vi "read can fd.vi"(8 "error in (no error)":errorcluster, 11 "channel":u16 format="%x") -> (0 "error out":errorcluster, 2 "queue empty?":bool, 3 "message":T5 {"id" format="%x"; "data" format="%x"}, 5 "ecc register":T1)   [LabVIEW 2024, in "atsj peakcan basic.lvlib"]
doc: "Reads a CAN FD message from the receive queue of an FD-capable PeakCAN <b>channel</b>."
uses:
  atsj peakcan basic.lvlib
  message type.ctl
  message.ctl
  support/x64/PCANBasic.dll
  ecc register error code.ctl
  ecc register direction.ctl
  ecc register segment.ctl
  ecc register.ctl
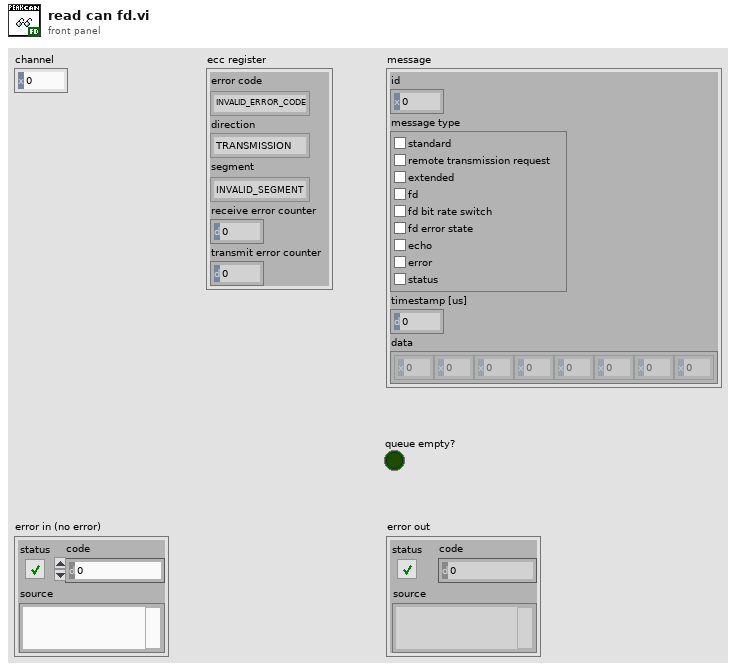
[diagram p1: front panel]
types:
  T1 = typedef "atsj peakcan basic.lvlib/ecc register.ctl" = cluster{"error code":T2, "direction":T3, "segment":T4, "receive error counter":u8, "transmit error counter":u8}
  T2 = typedef "atsj peakcan basic.lvlib/ecc register error code.ctl" = enum8{"INVALID_ERROR_CODE", "COUNTERS_UPDATE", "BIT_ERROR", "FORM_ERROR", "STUFF_ERROR", "OTHER_ERROR"}
  T3 = typedef "atsj peakcan basic.lvlib/ecc register direction.ctl" = enum16{"TRANSMISSION", "RECEPTION"}
  T4 = typedef "atsj peakcan basic.lvlib/ecc register segment.ctl" = enum8{"INVALID_SEGMENT", "ID_28_TO_ID_21", "START_OF_FRAME", "BIT_SRTR", "BIT_IDE", "ID_20_TO_ID_18", "ID_17_TO_ID_13", "CRC_SEQUENCE", "RESERVED_BIT_0", "DATA_FIELD", "DATA_LENGTH_CODE", "BIT_RTR", "RESERVED_BIT_1", "ID_4_TO_ID_0", "ID_12_TO_ID_5", "ACTIVE_ERROR_FLAG", "INTERMISSION", "TOLERATE_DOMINANT_BITS", "ERROR_DELIMITER", "CRC_DELIMITER", "ACKNOWLEDGE_SLOT", "END_OF_FRAME", "ACKNOWLEDGE_LIMITER", "OVERLOAD_FLAG"}
  T5 = typedef "atsj peakcan basic.lvlib/message.ctl" = cluster{"id":u32, "message type":T6, "timestamp [us]":u64, "data":u8[]}
  T6 = typedef "atsj peakcan basic.lvlib/message type.ctl" = cluster{"standard":bool, "remote transmission request ":bool, "extended":bool, "fd":bool, "fd bit rate switch":bool, "fd error state":bool, "echo":bool, "error":bool, "status":bool}
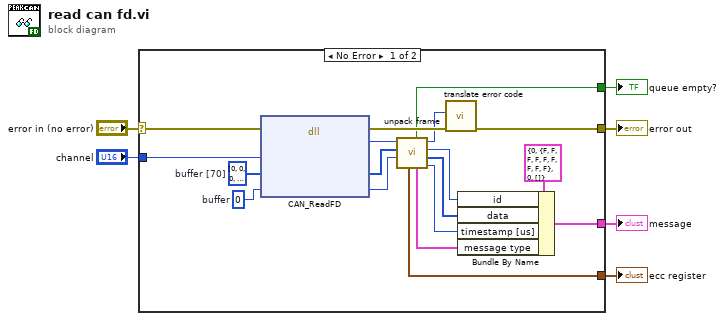
[diagram p0: block diagram]
diagram:
  n1 = case shown="No Error" "error in (no error)" {
    selector: "error in (no error)" -> [w18 w25]
    tunnel: [w11 w25] -> w5
    tunnel: "channel" -> [w12 _]
    tunnel: [w21 _] -> w3
    tunnel: [w19 _] -> w2
    tunnel: [w13 _] -> w1
    frame No Error {
      w7 = u8[] [0, 0, 0, 0, 0, 0, 0, 0, 0, 0, 0, 0, 0, 0, 0, 0, 0, 0, 0, 0, 0, 0, 0, 0, 0, 0, 0, 0, 0, 0, 0, 0, 0, 0, 0, 0, 0, 0, 0, 0, 0, 0, 0, 0, 0, 0, 0, 0, 0, 0, 0, 0, 0, 0, 0, 0, 0, 0, 0, 0, 0, 0, 0, 0, 0, 0, 0, 0, 0, 0]  # buffer [70]
      w23 = u64 0  # buffer
      n2 = dll-call lib="C:/atsj/plateau/atsj-peakcan-basic-for-labview/src/support/x64/PCANBasic.dll" fn="CAN_ReadFD" ("read can fd")(error in=w18, "Channel"=w12, "MessageBuffer"=w7, "TimestampBuffer"=w23) -> (error out=w24:errorcluster, "Status"=w20:u32, "MessageBuffer"=w10:u8[], "TimestampBuffer"=w9:u64)  [unwired: 3 in, 1 out]
      n3 = call "unpack frame.vi"("timestamp in"=w9, "frame"=w10, "status in"=w20) -> ("timestamp out"=w15:u64, "data"=w16:u8[], "id"=w17:u32, "status out"=w8:u32, "message type"=w14:T6, "queue empty?"=w19:bool, "ecc register"=w13:T1)  [unwired: 2 in]
      n4 = call "translate error code.vi"("error in (no error)"=w24, "error code"=w8) -> ("error out"=w11:errorcluster)  [unwired: 9 in]
      n5 = Bundle By Name(cluster=T5 {"id"=0, "message type"={"standard"=FALSE, "remote transmission request "=FALSE, "extended"=FALSE, "fd"=FALSE, "fd bit rate switch"=FALSE, "fd error state"=FALSE, "echo"=FALSE, "error"=FALSE, "status"=FALSE}, "timestamp [us]"=0, "data"=[]} ("message"), "id"=w17, "data"=w16, "timestamp [us]"=w15, "message type"=w14) -> (w21:T5)
    }
    frame Error {
    }
  }
  "error out" <- w5
  "message" <- w3
  "queue empty?" <- w2
  "ecc register" <- w1
